vi "get SPAN component params.vi"(8 "Fehler (Eingang)":errorcluster, 9 "Comp Idx":i32, 10 "active SPAN Idx":i32, 11 "SpanInletClusterArray":T4[](array[typedef]) {"zusätzliche Zeitdauer Erster Punkt" min=30 step=1 format="%#_5g"; "Zeitdauer Stufen" format="%#_5g"; "Max Fehler" format="%#_5g"; "Anzahl Stufen" format="%#_5g"; "Komponenten"."Komponente 5"."Komponente:" items=["NO (350,3000) LP 191C", "NO2 (150) LP 191C (1of2)", "NO2 (2000) LP 191C (2of2)", "N2O (300) LP 191C (1of2)", "NH3 (300) LP 191C (1of2)", "NH3 (900,3000) LP 191C (2of2)", "HNCO (400) 191C", "H2O% (30) LP 191C", "Formaldehyde (70,500) LP 191C", "CO2 low% (4) LP 191C (2of2)", "CO2% (20) LP 191C (1of2)", "CO (700) LP 191C (1of3)", "CO% (1) LP 191C (2of3)", "Propylene (1000) LP 191C", "Aromatic HC C7 (500) LP 191C", "Ethylene (1000) LP 191C", "CH4 (250) LP 191C (1of2)", "CH4 (5000) LP 191C (2of2)", "Ethane (1000) LP 191C", "Acetylene (1000) LP 191C", "HNO2 (20) 191C", "MeOH (1000) 191C", "CO% (10) LP 191C (3of3)", "Formic Acid (100) 191C", "SO2 (500) LP 191C", "Acetaldehyde (1000) LP 191C", "COS (100) LP 191C", "1,3 butadiene (100) LP 191C", "Oil as Octane (200) LP 191C", "N2O (1000) LP 191C (2of2)", "Propane (200) LP 191C", "NO2 autorange (2000)", "CO autorange (100000)", "CH4 autorange (5000)", "NH3 autorange (3000)", "Temp. Gascell", "Pressure Gascell", "sBeam@2500"]; "Komponenten"."Komponente 5"."Konzentration IST" format="%#.4f"; "Komponenten"."Komponente 5"."Genauigkeit" format="%#.1f"; "Komponenten"."Komponente 4"."Komponente:" items=["NO (350,3000) LP 191C", "NO2 (150) LP 191C (1of2)", "NO2 (2000) LP 191C (2of2)", "N2O (300) LP 191C (1of2)", "NH3 (300) LP 191C (1of2)", "NH3 (900,3000) LP 191C (2of2)", "HNCO (400) 191C", "H2O% (30) LP 191C", "Formaldehyde (70,500) LP 191C", "CO2 low% (4) LP 191C (2of2)", "CO2% (20) LP 191C (1of2)", "CO (700) LP 191C (1of3)", "CO% (1) LP 191C (2of3)", "Propylene (1000) LP 191C", "Aromatic HC C7 (500) LP 191C", "Ethylene (1000) LP 191C", "CH4 (250) LP 191C (1of2)", "CH4 (5000) LP 191C (2of2)", "Ethane (1000) LP 191C", "Acetylene (1000) LP 191C", "HNO2 (20) 191C", "MeOH (1000) 191C", "CO% (10) LP 191C (3of3)", "Formic Acid (100) 191C", "SO2 (500) LP 191C", "Acetaldehyde (1000) LP 191C", "COS (100) LP 191C", "1,3 butadiene (100) LP 191C", "Oil as Octane (200) LP 191C", "N2O (1000) LP 191C (2of2)", "Propane (200) LP 191C", "NO2 autorange (2000)", "CO autorange (100000)", "CH4 autorange (5000)", "NH3 autorange (3000)", "Temp. Gascell", "Pressure Gascell", "sBeam@2500"]; "Komponenten"."Komponente 4"."Konzentration IST" format="%#.4f"; "Komponenten"."Komponente 4"."Genauigkeit" format="%#.1f"; "Komponenten"."Komponente 3"."Komponente:" items=["NO (350,3000) LP 191C", "NO2 (150) LP 191C (1of2)", "NO2 (2000) LP 191C (2of2)", "N2O (300) LP 191C (1of2)", "NH3 (300) LP 191C (1of2)", "NH3 (900,3000) LP 191C (2of2)", "HNCO (400) 191C", "H2O% (30) LP 191C", "Formaldehyde (70,500) LP 191C", "CO2 low% (4) LP 191C (2of2)", "CO2% (20) LP 191C (1of2)", "CO (700) LP 191C (1of3)", "CO% (1) LP 191C (2of3)", "Propylene (1000) LP 191C", "Aromatic HC C7 (500) LP 191C", "Ethylene (1000) LP 191C", "CH4 (250) LP 191C (1of2)", "CH4 (5000) LP 191C (2of2)", "Ethane (1000) LP 191C", "Acetylene (1000) LP 191C", "HNO2 (20) 191C", "MeOH (1000) 191C", "CO% (10) LP 191C (3of3)", "Formic Acid (100) 191C", "SO2 (500) LP 191C", "Acetaldehyde (1000) LP 191C", "COS (100) LP 191C", "1,3 butadiene (100) LP 191C", "Oil as Octane (200) LP 191C", "N2O (1000) LP 191C (2of2)", "Propane (200) LP 191C", "NO2 autorange (2000)", "CO autorange (100000)", "CH4 autorange (5000)", "NH3 autorange (3000)", "Temp. Gascell", "Pressure Gascell", "sBeam@2500"]; "Komponenten"."Komponente 3"."Konzentration IST" format="%#.4f"; "Komponenten"."Komponente 3"."Genauigkeit" format="%#.1f"; "Komponenten"."Komponente 2"."Komponente:" items=["NO (350,3000) LP 191C", "NO2 (150) LP 191C (1of2)", "NO2 (2000) LP 191C (2of2)", "N2O (300) LP 191C (1of2)", "NH3 (300) LP 191C (1of2)", "NH3 (900,3000) LP 191C (2of2)", "HNCO (400) 191C", "H2O% (30) LP 191C", "Formaldehyde (70,500) LP 191C", "CO2 low% (4) LP 191C (2of2)", "CO2% (20) LP 191C (1of2)", "CO (700) LP 191C (1of3)", "CO% (1) LP 191C (2of3)", "Propylene (1000) LP 191C", "Aromatic HC C7 (500) LP 191C", "Ethylene (1000) LP 191C", "CH4 (250) LP 191C (1of2)", "CH4 (5000) LP 191C (2of2)", "Ethane (1000) LP 191C", "Acetylene (1000) LP 191C", "HNO2 (20) 191C", "MeOH (1000) 191C", "CO% (10) LP 191C (3of3)", "Formic Acid (100) 191C", "SO2 (500) LP 191C", "Acetaldehyde (1000) LP 191C", "COS (100) LP 191C", "1,3 butadiene (100) LP 191C", "Oil as Octane (200) LP 191C", "N2O (1000) LP 191C (2of2)", "Propane (200) LP 191C", "NO2 autorange (2000)", "CO autorange (100000)", "CH4 autorange (5000)", "NH3 autorange (3000)", "Temp. Gascell", "Pressure Gascell", "sBeam@2500"]; "Komponenten"."Komponente 2"."Konzentration IST" format="%#.4f"; "Komponenten"."Komponente 2"."Genauigkeit" format="%#.1f"; "Komponenten"."Komponente 1"."Komponente:" items=["NO (350,3000) LP 191C", "NO2 (150) LP 191C (1of2)", "NO2 (2000) LP 191C (2of2)", "N2O (300) LP 191C (1of2)", "NH3 (300) LP 191C (1of2)", "NH3 (900,3000) LP 191C (2of2)", "HNCO (400) 191C", "H2O% (30) LP 191C", "Formaldehyde (70,500) LP 191C", "CO2 low% (4) LP 191C (2of2)", "CO2% (20) LP 191C (1of2)", "CO (700) LP 191C (1of3)", "CO% (1) LP 191C (2of3)", "Propylene (1000) LP 191C", "Aromatic HC C7 (500) LP 191C", "Ethylene (1000) LP 191C", "CH4 (250) LP 191C (1of2)", "CH4 (5000) LP 191C (2of2)", "Ethane (1000) LP 191C", "Acetylene (1000) LP 191C", "HNO2 (20) 191C", "MeOH (1000) 191C", "CO% (10) LP 191C (3of3)", "Formic Acid (100) 191C", "SO2 (500) LP 191C", "Acetaldehyde (1000) LP 191C", "COS (100) LP 191C", "1,3 butadiene (100) LP 191C", "Oil as Octane (200) LP 191C", "N2O (1000) LP 191C (2of2)", "Propane (200) LP 191C", "NO2 autorange (2000)", "CO autorange (100000)", "CH4 autorange (5000)", "NH3 autorange (3000)", "Temp. Gascell", "Pressure Gascell", "sBeam@2500"]; "Komponenten"."Komponente 1"."Konzentration IST" format="%#.4f"; "Komponenten"."Komponente 1"."Genauigkeit" format="%#.1f"; "Ablaufdatum" format="%<%d.%m.%Y>T"; "Gasflasche" items=["----"=10000, "IAG NH3 3000"=0, "IAG NH3 200"=1, "IAG NH3 2000"=2, "IAG MG"=3, "IAG O2"=4]}) -> (0 "Fehler (Ausgang)":errorcluster, 3 "Component Cluster":T3={"Component"={"Component Name"="", "Component"=0, "Component Unit"=""}, "Daten aufzeichnen Offset Cluster"={"Autorange Offsets"="", "Autorange Spanfactors"="", "Polynome"={"Polynome[0]"=0.0, "Polynome[1]"=0.0, "Polynome[2]"=0.0, "Polynome[3]"=0.0, "Polynome[4]"=0.0}}, "Lin Offset Cluster"={"Autorange Offsets"="", "Autorange Spanfactors"="", "Polynome"={"Polynome[0]"=0.0, "Polynome[1]"=0.0, "Polynome[2]"=0.0, "Polynome[3]"=0.0, "Polynome[4]"=0.0}, "Polynom-Ordnung"=enum."autom."}, "EPA Optionsfeld"=enum."Rohwert"})   [LabVIEW 2020, in "Linearisierung v2.lvlib" / "Gasteiler.lvlib"]
uses:
  Gasteiler/Gasteiler.lvlib
  SpanInletCluster.ctl
  Seiten/System Einstellungen V2/Konfig Gasflasche.ctl
  Seiten/System Einstellungen V2/Analysatoren.ctl
  Seiten/System Einstellungen V2/Gasflasche Auswahl.ctl
  Komponentencluster mit Formel.ctl
  Komponentenauswahl mit Formel.ctl
  Visualisierungs Elemente/String - Eingabefeld.ctl
  Einheit.ctl
  Seiten/System Einstellungen V2/Traegergas.ctl
  Auswahl Polynom Ordnung.ctl
  EPA Optionsfeld.ctl
  Lin-Polynom Daten.ctl
  KomponentenArray.ctl
  Visualisierungs Elemente/Auswahlfeld.ctl
  Visualisierungs Elemente/Zahlen-Eingabefeld.ctl
  Gasteiler/HovaCal/AutoLin Hovacal.ctl
  Kalibrieroption.ctl
  EPA1065-307/Condition.ctl
  Gasteiler/HovaCAL_Interface/Controls/Flow Einstellung.ctl
  Gasteiler/HovaCAL_Interface/Controls/Pump state.ctl
  Seiten/CalGas Aufschaltung/Lin Modus.ctl
  SpanEinstellungen.lvlib
  Linearisierung v2.lvlib
  Protokoll/Protokoll.lvlib
  Gasteiler/HovaCal/HovaCal.lvlib
  EPA1065-307/Linearity verification 1065-307.lvlib
  Seiten/System Einstellungen V2/System Einstellungen V2.lvlib
  Gasteiler/HovaCAL_Interface/Controls/Controls.lvlib
  Seiten/CalGas Aufschaltung/CalGas Aufschaltung.lvlib
panel:
  # "sec"
  # "%"
  # "sec"
  # "Komponente"
  # "Formel"
  # "Konzentration"
  # "Einheit"
  # "Genauigkeit [%]"
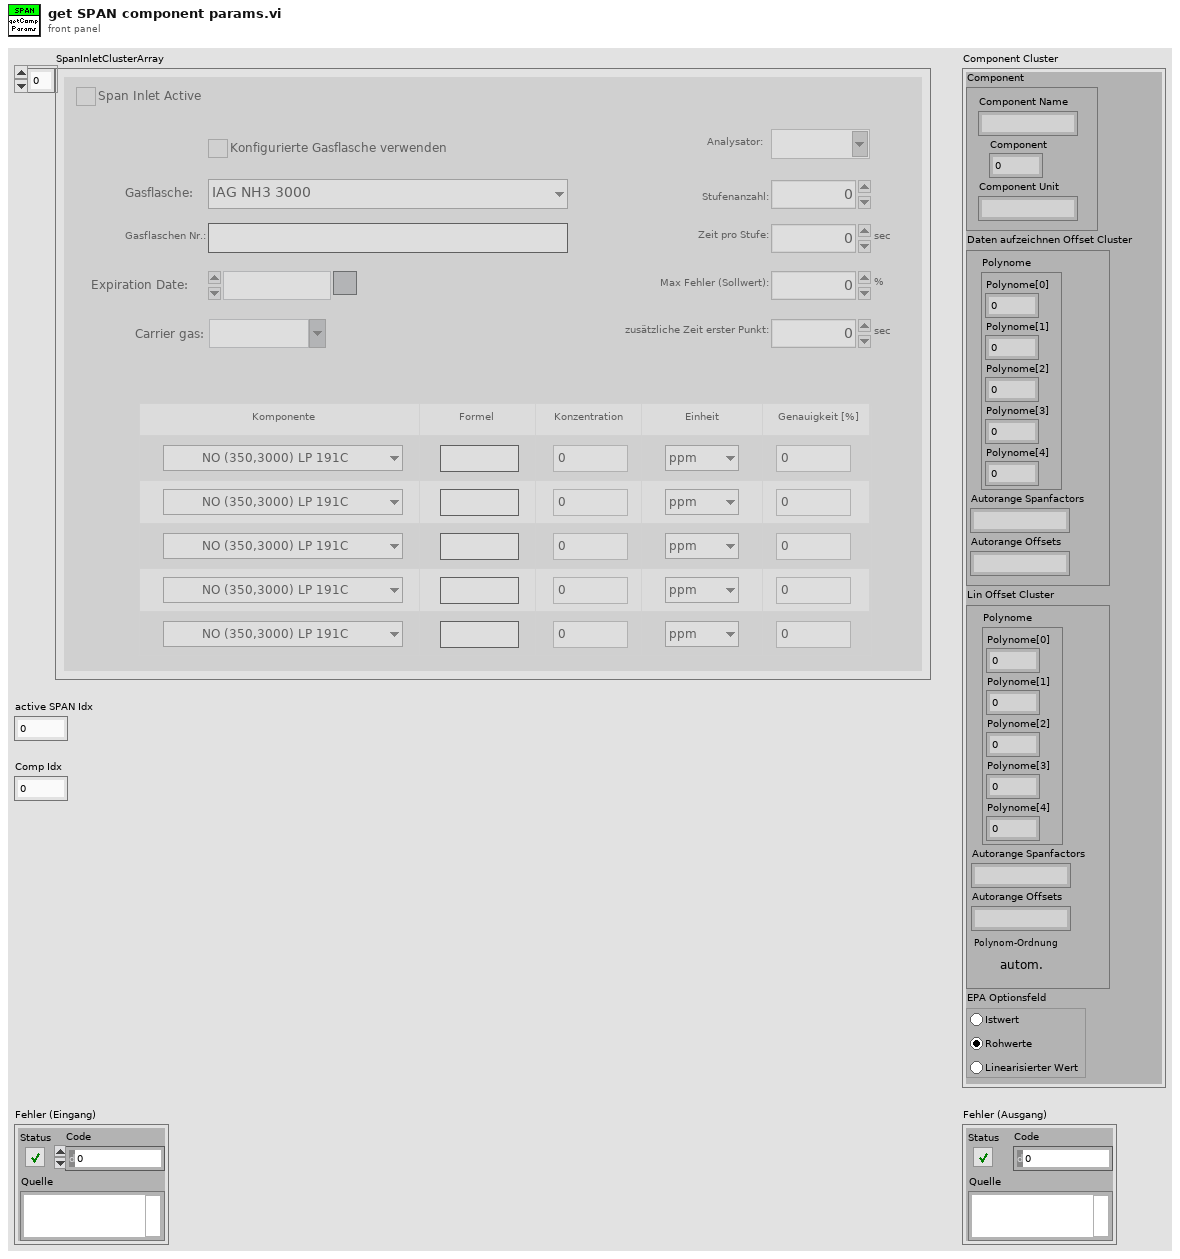
[diagram p1: front panel]
types:
  T1 = typedef "Linearisierung v2.lvlib/Auswahl Polynom Ordnung.ctl" = enum16{"autom.", "raw", "actual", "1", "2", "3", "4"}
  T2 = typedef "Linearisierung v2.lvlib/EPA Optionsfeld.ctl" = enum32{"Istwert", "Rohwert", "Linearisierter Wert"}
  T3 = cluster{"Component":cluster{"Component Name":string, "Component":u8, "Component Unit":string}, "Daten aufzeichnen Offset Cluster":cluster{"Autorange Offsets":string, "Autorange Spanfactors":string, "Polynome":cluster{"Polynome[0]":dbl, "Polynome[1]":dbl, "Polynome[2]":dbl, "Polynome[3]":dbl, "Polynome[4]":dbl}}, "Lin Offset Cluster":cluster{"Autorange Offsets":string, "Autorange Spanfactors":string, "Polynome":cluster{"Polynome[0]":dbl, "Polynome[1]":dbl, "Polynome[2]":dbl, "Polynome[3]":dbl, "Polynome[4]":dbl}, "Polynom-Ordnung":T1}, "EPA Optionsfeld":T2}
  T4 = typedef "Linearisierung v2.lvlib/SpanEinstellungen.lvlib/SpanInletCluster.ctl" = cluster{"Span Inlet Active":T5, "Analysator":T6, "Konfig Gasflasche":T5, "Gasflasche":T7, "Gasflaschen Nr.:":string, "Ablaufdatum":timestamp, "Komponenten":T8, "Zeitdauer Stufen":sgl, "Max Fehler":sgl, "Anzahl Stufen":sgl, "Trägergas":T12, "zusätzliche Zeitdauer Erster Punkt":sgl}
  T5 = typedef "System Einstellungen V2.lvlib/Konfig Gasflasche.ctl" = bool
  T6 = typedef "System Einstellungen V2.lvlib/Analysatoren.ctl" = string
  T7 = typedef "System Einstellungen V2.lvlib/Gasflasche Auswahl.ctl" = u16
  T8 = typedef "Linearisierung v2.lvlib/SpanEinstellungen.lvlib/Komponentencluster mit Formel.ctl" = cluster{"Komponente 1":T9, "Komponente 2":T9, "Komponente 3":T9, "Komponente 4":T9, "Komponente 5":T9}
  T9 = typedef "Linearisierung v2.lvlib/SpanEinstellungen.lvlib/Komponentenauswahl mit Formel.ctl" = cluster{"Komponente:":u16, "Summenformel":T10, "Konzentration IST":dbl, "Einheit":T11, "Genauigkeit":dbl}
  T10 = typedef "String - Eingabefeld.ctl" = string
  T11 = typedef "Linearisierung v2.lvlib/SpanEinstellungen.lvlib/Einheit.ctl" = enum16{"ppm", "%"}
  T12 = typedef "System Einstellungen V2.lvlib/Traegergas.ctl" = string
  T13 = typedef "Linearisierung v2.lvlib/Protokoll.lvlib/Aktion LIN Polynom Ordnung je Komponente für Protokoll.ctl" = enum16{"lesen", "schreiben", "init", "schreiben viewonly", "init initial"}
  T14 = cluster{"Autorange Offsets":string, "Autorange Spanfactors":string, "Polynome":cluster{"Polynome[0]":dbl, "Polynome[1]":dbl, "Polynome[2]":dbl, "Polynome[3]":dbl, "Polynome[4]":dbl}, "Polynom-Ordnung":T1}
  T15 = cluster{"Autorange Offsets":string, "Autorange Spanfactors":string, "Polynome":cluster{"Polynome[0]":dbl, "Polynome[1]":dbl, "Polynome[2]":dbl, "Polynome[3]":dbl, "Polynome[4]":dbl}}
  T16 = typedef "Linearisierung v2.lvlib/Lin-Polynom Daten.ctl" = cluster{"Messgerät":string, "Kalibrator (Gasteiler)":string, "Bearbeiter/in":string, "Komponente":string, "Zeitstempel":timestamp, "F_max gefordert (%)":sgl, "F_max in %":sgl, "F_max in ppm":sgl, "Vorschlag Ordnung":i32, "Polynom OK":bool, "Polynomkoeff.":dbl[], "Prüfgas Konzentration":dbl, "Pfad EPA":string, "Pfad_LIN":string, "Gasnummer:":u8, "Komponentenauswahl":T17, "Verdünnungsgas":T19, "Zeitdauer Stufe":T20, "Anzahl Stufen":T20, "F_max in % EPA":sgl, "F_max in ppm EPA":sgl, "F_max in % LIN":sgl, "F_max in ppm LIN":sgl, "Punkte umkehren":bool, "EPA Optionsfeld":T2, "Autolin Hovacal":T21, "Spanfactors":sgl[], "Kalibrierauswahl":T22, "Conditions:":T23, "Gasflaschen Nr.:":string, "Bottle Accuracy":dbl, "Konfig Gasflasche":T5, "Gasflasche":T7, "HovaCAL Flow AutoLin":T24, "MFC Output":T25, "Gas Ablaufdatum":timestamp, "Lin Modus":T26, "zusätzliche Zeitdauer Erster Punkt":sgl, "Offsets":sgl[]}
  T17 = typedef "Linearisierung v2.lvlib/KomponentenArray.ctl" = cluster{"Komponente:":T18, "Konzentration":dbl}[]
  T18 = typedef "Auswahlfeld.ctl" = u16
  T19 = typedef "Linearisierung v2.lvlib/Gasteiler.lvlib/Prüfgas in.ctl" = u16
  T20 = typedef "Zahlen-Eingabefeld.ctl" = sgl
  T21 = typedef "Linearisierung v2.lvlib/Gasteiler.lvlib/HovaCal.lvlib/AutoLin Hovacal.ctl" = enum32{"Keine Auswahl", "Optionsauswahl 1", "Optionsauswahl 2"}
  T22 = typedef "Linearisierung v2.lvlib/Kalibrieroption.ctl" = u16
  T23 = typedef "Linearisierung v2.lvlib/Linearity verification 1065-307.lvlib/Condition.ctl" = u16
  T24 = typedef "Linearisierung v2.lvlib/Gasteiler.lvlib/HovaCAL_Interface.lvlib/Controls.lvlib/Flow Einstellung.ctl" = cluster{"HovaCAL Flow Input Cluster":dbl}
  T25 = typedef "Linearisierung v2.lvlib/Gasteiler.lvlib/HovaCAL_Interface.lvlib/Controls.lvlib/Pump state.ctl" = cluster{"Run":bool}
  T26 = typedef "CalGas Aufschaltung.lvlib/Lin Modus.ctl" = u16
  T27 = typedef "Linearisierung v2.lvlib/Protokoll.lvlib/Aktion EPA Polynom Ordnung je Komponente für Protokoll.ctl" = enum16{"lesen", "schreiben", "init", "init initial"}
  T28 = typedef "String - Ausgabefeld.ctl" = string
  T29 = cluster{"Component Name":T28, "Compnent Nr":u16, "Formelname(n)":string}
  T30 = cluster{"Polynome[0]":dbl, "Polynome[1]":dbl, "Polynome[2]":dbl, "Polynome[3]":dbl, "Polynome[4]":dbl}
  T31 = cluster{"Component Name":T28, i32, "Einheit in String":string}
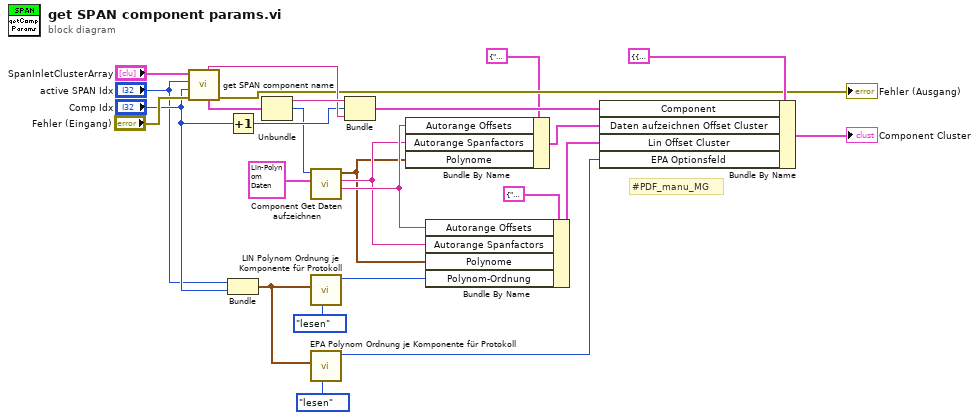
[diagram p0: block diagram]
diagram:
  # "#PDF_manu_MG"
  n1 = call "get SPAN component name.vi"("Fehler (Eingang)"="Fehler (Eingang)", "Comp Idx"="Comp Idx", "SPAN Idx"="active SPAN Idx", "SpanInletClusterArray in"="SpanInletClusterArray") -> ("Fehler (Ausgang)"=→"Fehler (Ausgang)":errorcluster, "Komponente Nr Name -Cluster"=w23:T29, "Einheit in String"=w25:string)  [unwired: 5 out]
  n2 = Increment(x="Comp Idx") -> (x+1=w24:i32)
  n3 = Bundle("active SPAN Idx"="active SPAN Idx", "Comp Idx"="Comp Idx") -> (w1:cluster{"active SPAN Idx":i32, "Comp Idx":i32})  [unwired: 1 in]
  n4 = Unbundle(w23) -> ("Component Name"=w26:T28, "Compnent Nr"=w17:u16)  [unwired: 1 out]
  n5 = call "Component Get Daten aufzeichnen.vi"("Lin-Polynom"=T16 {"Messgerät"="", "Kalibrator (Gasteiler)"="", "Bearbeiter/in"="", "Komponente"="", "Zeitstempel"=timestamp(0 s since 1904-01-01), "F_max gefordert (%)"=0.0, "F_max in %"=0.0, "F_max in ppm"=0.0, "Vorschlag Ordnung"=0, "Polynom OK"=FALSE, "Polynomkoeff."=[], "Prüfgas Konzentration"=0.0, "Pfad EPA"="", "Pfad_LIN"="", "Gasnummer:"=0, "Komponentenauswahl"=[], "Verdünnungsgas"=0, "Zeitdauer Stufe"=0.0, "Anzahl Stufen"=0.0, "F_max in % EPA"=0.0, "F_max in ppm EPA"=0.0, "F_max in % LIN"=0.0, "F_max in ppm LIN"=0.0, "Punkte umkehren"=FALSE, "EPA Optionsfeld"=enum."Istwert", "Autolin Hovacal"=enum."Keine Auswahl", "Spanfactors"=[], "Kalibrierauswahl"=0, "Conditions:"=0, "Gasflaschen Nr.:"="", "Bottle Accuracy"=0.0, "Konfig Gasflasche"=FALSE, "Gasflasche"=0, "HovaCAL Flow AutoLin"={"HovaCAL Flow Input Cluster"=0.0}, "MFC Output"={"Run"=FALSE}, "Gas Ablaufdatum"=timestamp(0 s since 1904-01-01), "Lin Modus"=0, "zusätzliche Zeitdauer Erster Punkt"=0.0, "Offsets"=[]}, "Gaskomponente"=w17) -> ("Autorange Offsets"=w8:string, "Autorange Spanfactors"=w7:string, "Polynome"=w6:T30)  [unwired: 6 in, 1 out]
  n6 = call "LIN Polynom Ordnung je Komponente für Protokoll.vi"("Aktion"=Aktion_LIN_Polynom_Ordnung_je_Komponente_für_Protokoll."lesen", "Index in"=w1) -> ("Polynom-Ordnung out"=w5:T1)  [unwired: 3 in, 6 out]
  n7 = call "EPA Polynom Ordnung je Komponente für Protokoll.vi"("Aktion"=Aktion_EPA_Polynom_Ordnung_je_Komponente_für_Protokoll."lesen", "Index in"=w1) -> ("EPA Optionsfeld out"=w4:T2)  [unwired: 5 in, 3 out]
  n8 = Bundle("Component Name"=w26, w24, "Einheit in String"=w25) -> (w20:T31)  [unwired: 1 in]
  n9 = Bundle By Name(cluster=T15 {"Autorange Offsets"="", "Autorange Spanfactors"="", "Polynome"={"Polynome[0]"=0.0, "Polynome[1]"=0.0, "Polynome[2]"=0.0, "Polynome[3]"=0.0, "Polynome[4]"=0.0}} ("Daten aufzeichnen Offset Cluster"), "Autorange Offsets"=w8, "Autorange Spanfactors"=w7, "Polynome"=w6) -> (w11:T15)
  n10 = Bundle By Name(cluster=T14 {"Autorange Offsets"="", "Autorange Spanfactors"="", "Polynome"={"Polynome[0]"=0.0, "Polynome[1]"=0.0, "Polynome[2]"=0.0, "Polynome[3]"=0.0, "Polynome[4]"=0.0}, "Polynom-Ordnung"=enum."autom."} ("Lin Offset Cluster"), "Autorange Offsets"=w8, "Autorange Spanfactors"=w7, "Polynome"=w6, "Polynom-Ordnung"=w5) -> (w9:T14)
  n11 = Bundle By Name(cluster=T3 {"Component"={"Component Name"="", "Component"=0, "Component Unit"=""}, "Daten aufzeichnen Offset Cluster"={"Autorange Offsets"="", "Autorange Spanfactors"="", "Polynome"={"Polynome[0]"=0.0, "Polynome[1]"=0.0, "Polynome[2]"=0.0, "Polynome[3]"=0.0, "Polynome[4]"=0.0}}, "Lin Offset Cluster"={"Autorange Offsets"="", "Autorange Spanfactors"="", "Polynome"={"Polynome[0]"=0.0, "Polynome[1]"=0.0, "Polynome[2]"=0.0, "Polynome[3]"=0.0, "Polynome[4]"=0.0}, "Polynom-Ordnung"=enum."autom."}, "EPA Optionsfeld"=enum."Rohwert"} ("Component Cluster"), "Component"=w20, "Daten aufzeichnen Offset Cluster"=w11, "Lin Offset Cluster"=w9, "EPA Optionsfeld"=w4) -> (→"Component Cluster":T3)
